vi "Generate MCM Signals.vi"(4 "noise amplitude":dbl=0.01 format="%.2f", 5 "Add Noise?":bool, 6 "sampling info":cluster{"Fs":dbl, "#s":dbl}={"Fs"=1000.0, "#s"=1000.0} {"Fs" format="%.2p"}, 7 "Reset":bool, 8 "error in":errorcluster, 9 "square wave duty cycle (%)":dbl=50.0, 10 "Vibration":T1(array[cluster]), 11 "Tachometer":cluster{"RPM":sgl}={"RPM"=60.0} {"RPM" scale=1.0..6000.0}) -> (0 "error out":errorcluster, 2 "Vibration signals":waveform(dbl)[](array[waveform]), 3 "Tach signal":waveform(dbl))   [LabVIEW 2017, in "CmsAcquisition.lvlib"]
uses:
  <vilib>/addons/InsightCM/Devices/Shared/Cms/CmsAcquisition/CmsAcquisition.lvlib
  <vilib>/measure/NI_MABase.lvlib
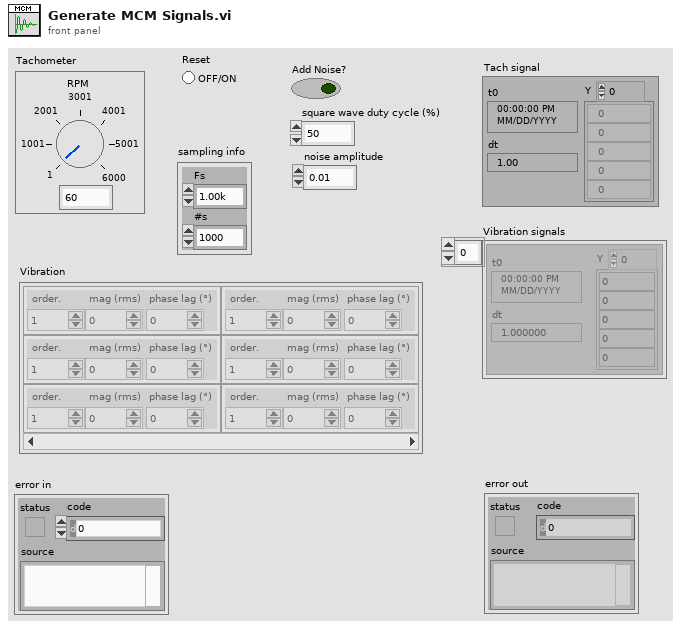
[diagram p1: front panel]
types:
  T1 = cluster{"order.":dbl, "mag (rms)":dbl, "phase lag (°)":dbl}[][]
  T2 = enum16{"Sine Wave", "Triangle Wave", "Square Wave", "Sawtooth Wave"}
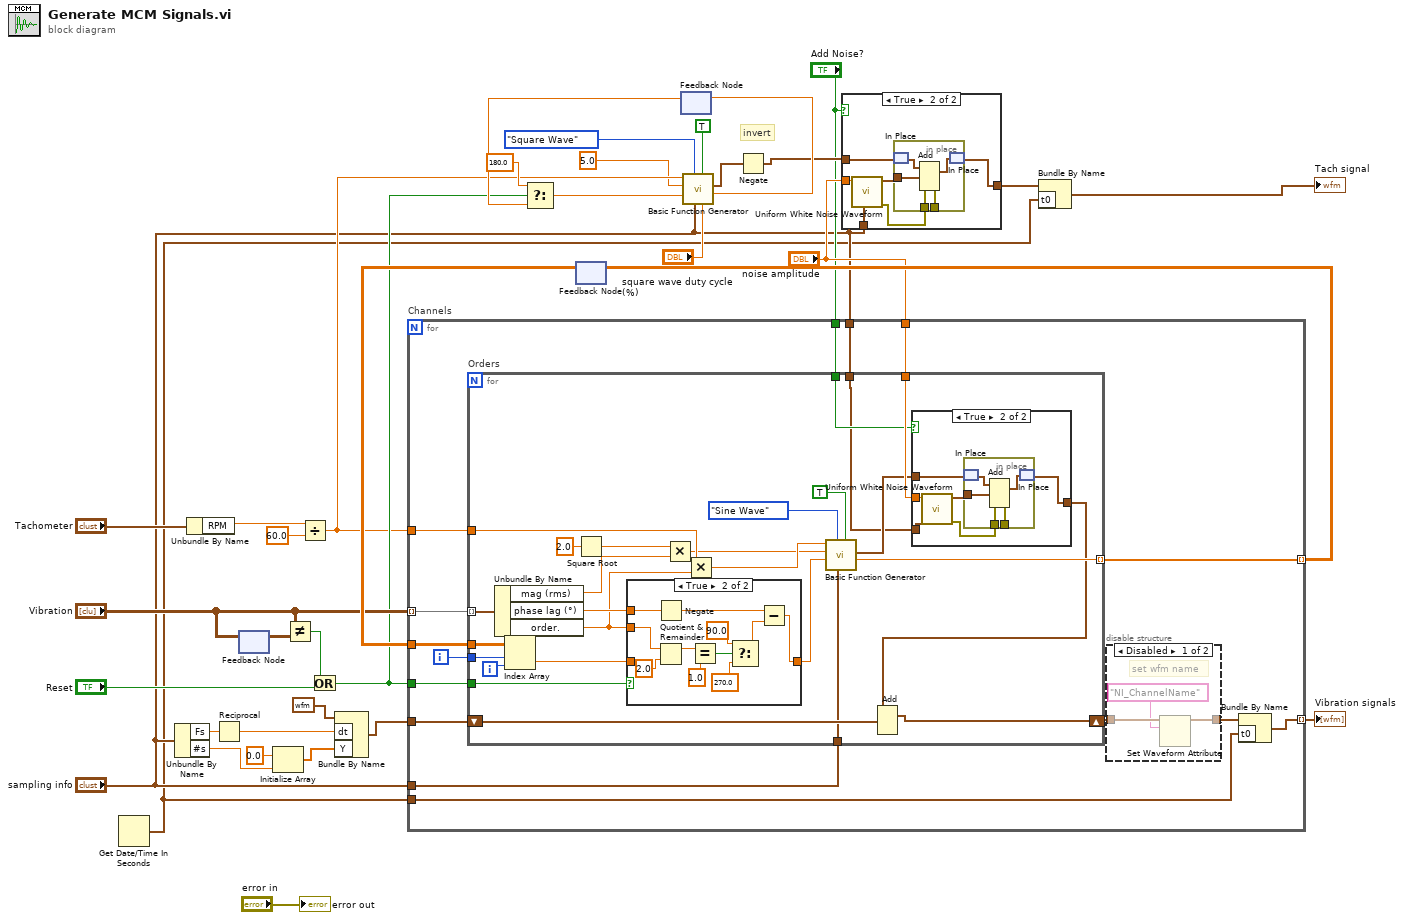
[diagram p0: block diagram]
diagram:
  # "invert"
  n1 = Get Date/Time In Seconds() -> (seconds since 1Jan1904=w1:timestamp)
  n2 = Unbundle By Name("sampling info") -> ("Fs"=w27:dbl, "#s"=w25:dbl)
  n3 = Unbundle By Name("Tachometer") -> ("RPM"=w21:sgl)
  n4 = Reciprocal(x=w27) -> (1/x=w26:dbl)
  n5 = feedback #1() -> (w35:T1)  [unwired: 1 in]
  n6 = feedback-in #1("Vibration") -> ()
  n7 = Initialize Array(0.0 ("element"), w25) -> (w24:dbl[])
  n8 = Not Equal?(x="Vibration", y=w35) -> (x != y?=w34:bool)
  n9 = Divide(x=w21, y=sgl 60.0) -> (x/y=w10:sgl)
  n10 = Or(x=w34, y="Reset") -> (x .or. y?=w11:bool)
  n11 = Bundle By Name(cluster=waveform(dbl) {"t0"=timestamp(0 s since 1904-01-01), "dt"=1.0, "Y"=[]} ("signal out"), "dt"=w26, "Y"=w24) -> (w28:waveform(dbl))
  n12 = feedback #2() -> (w32:dbl[][])  [unwired: 1 in]
  n13 = for "Channels" {
    tunnel: [w51] -> w33 mode=indexing
    tunnel: "Vibration" -> [w50] mode=indexing
    tunnel: w32 -> [w49]
    tunnel: w11 -> [w48]
    tunnel: [w39] -> w30 mode=indexing
    tunnel: "sampling info" -> [w47]
    tunnel: w10 -> [w46]
    tunnel: w28 -> [w45]
    tunnel: "noise amplitude" -> [w42]
    tunnel: "Add Noise?" -> [w41]
    tunnel: "sampling info" -> [w40]
    tunnel: w1 -> [w37]
    i -> [w44]
    n14 = for "Orders" {
      shift-right: [w70] -> w43
      shift-left: w45 -> [w81]
      tunnel: [w75] -> w51 mode=indexing
      tunnel: w50 -> [w80] mode=indexing
      tunnel: w49 -> [w77]
      tunnel: w48 -> [w64]
      tunnel: w44 -> [w79]
      tunnel: w47 -> [w73]
      tunnel: w46 -> [w72]
      tunnel: w42 -> [w60]
      tunnel: w41 -> [w59]
      tunnel: w40 -> [w56]
      i -> [w78]
      n15 = Unbundle By Name(w80) -> ("mag (rms)"=w68:dbl, "phase lag (°)"=w65:dbl, "order."=w61:dbl)
      n16 = Index Array(array=w77, index (row)=w79, index (col)=w78) -> (element=w63:dbl)
      n17 = Square Root(x=2.0) -> (sqrt(x)=w67:dbl)
      n18 = case shown="True" w64 {
        tunnel: w65 -> [_ w96]
        tunnel: w63 -> [w94 _]
        tunnel: [w94 w100] -> w62
        tunnel: w61 -> [_ w105]
        frame False {
        }
        frame True {
          n19 = Negate(x=w96) -> (-x=w95:dbl)
          n20 = Quotient & Remainder(x=w105, y=2.0) -> (x-y*floor(x/y)=w103:dbl)  [unwired: 1 out]
          n21 = Equal?(x=w103, y=1.0) -> (x = y?=w101:bool)
          n22 = Select(t=90.0, s=w101, f=270.0) -> (s? t:f=w99:dbl)
          n23 = Subtract(x=w95, y=w99) -> (x-y=w100:dbl)
        }
      }
      n24 = Multiply(x=w67, y=w68) -> (x*y=w69:dbl)
      n25 = Multiply(x=w72, y=w61) -> (x*y=w71:dbl)
      n26 = call <vilib>:"Basic Function Generator.vi"("reset signal"=TRUE ("reset phase"), "sampling info"=w73, "signal type"=T2."Sine Wave", "phase"=w62, "amplitude"=w69, "frequency"=w71) -> ("phase out"=w75:dbl, "signal out"=w58:waveform(dbl))  [unwired: 3 in, 1 out]
      n27 = case shown="True" w59 {
        tunnel: w60 -> [_ w88]
        tunnel: [w82 w87] -> w57
        tunnel: w56 -> [_ w86]
        tunnel: w58 -> [w82 w84]
        frame False {
        }
        frame True {
          n28 = call <vilib>:"Uniform White Noise Waveform.vi"("sampling info"=w86, "amplitude"=w88) -> ("error out"=w83:errorcluster, "signal out"=w85:waveform(dbl))  [unwired: 8 in]
          n29 = in-place {
            in-place-border: w83 -> [w92]
            in-place-border: [w91] -> _
            in-place-border: w85 -> [w89]
            n30 = in-place-match #3(w84) -> (w93:waveform(dbl))
            n31 = Add(1:w89, 2:w93, 4:w92) -> (0:w90:waveform(dbl), 3:w91:errorcluster)
            n32 = in-place-match #3(w90) -> (w87:waveform(dbl))
          }
        }
      }
      n33 = Add(1:w81, 2:w57) -> (0:w70:waveform(dbl))  [unwired: 1 in, 1 out]
    }
    n34 = disable-structure shown="Disabled" {
      disable-tunnel: w43 -> [w54 w55]
      disable-tunnel: [w53 w55] -> w38
      frame Disabled {
        # "set wfm name"
        n35 = Set Waveform Attribute(6:"NI_ChannelName" ("name"), 7:w54) -> (3:w53:waveform(dbl))  [unwired: 2 in, 2 out]
      }
      frame Enabled {
      }
    }
    n36 = Bundle By Name(cluster=w38, "t0"=w37) -> (w39:waveform(dbl))
  }
  "Vibration signals" <- w30
  n37 = feedback-in #2(w33) -> ()
  n38 = feedback #4() -> (w13:dbl)  [unwired: 1 in]
  n39 = Select(t=180.0, s=w11, f=w13) -> (s? t:f=w14:dbl)
  n40 = call <vilib>:"Basic Function Generator.vi"("square wave duty cycle (%)"="square wave duty cycle (%)", "reset signal"=TRUE, "sampling info"="sampling info", "signal type"=T2."Square Wave", "phase"=w14, "amplitude"=5.0, "frequency"=w10) -> ("phase out"=w18:dbl, "signal out"=w9:waveform(dbl))  [unwired: 2 in, 1 out]
  n41 = feedback-in #4(w18) -> ()
  n42 = Negate(x=w9) -> (-x=w7:waveform(dbl))
  n43 = case shown="True" "Add Noise?" {
    tunnel: "noise amplitude" -> [_ w112]
    tunnel: [w106 w111] -> w2
    tunnel: "sampling info" -> [_ w110]
    tunnel: w7 -> [w106 w108]
    frame False {
    }
    frame True {
      n44 = call <vilib>:"Uniform White Noise Waveform.vi"("sampling info"=w110, "amplitude"=w112) -> ("error out"=w107:errorcluster, "signal out"=w109:waveform(dbl))  [unwired: 8 in]
      n45 = in-place {
        in-place-border: w107 -> [w116]
        in-place-border: [w115] -> _
        in-place-border: w109 -> [w113]
        n46 = in-place-match #5(w108) -> (w117:waveform(dbl))
        n47 = Add(1:w113, 2:w117, 4:w116) -> (0:w114:waveform(dbl), 3:w115:errorcluster)
        n48 = in-place-match #5(w114) -> (w111:waveform(dbl))
      }
    }
  }
  n49 = Bundle By Name(cluster=w2, "t0"=w1) -> (→"Tach signal":waveform(dbl))
  "error out" <- "error in"
